vi "limit_array_size.vi"(10 "max size":i32, 11 "dbl array in":dbl[](array[numeric])) -> (3 "dbl array out":dbl[](array[numeric]))   [LabVIEW 2011]
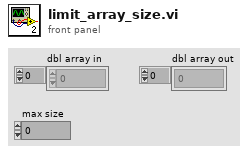
[diagram p1: front panel]
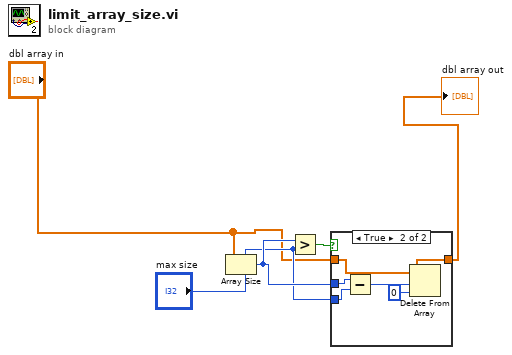
[diagram p0: block diagram]
diagram:
  n1 = Array Size(array="dbl array in") -> (size(s)=w5:i32)
  n2 = Greater?(x=w5, y="max size") -> (0:w1:bool)
  n3 = case shown="True" w1 {
    tunnel: "dbl array in" -> [w6 w12]
    tunnel: [w6 w11] -> w3
    tunnel: "max size" -> [_ w8]
    tunnel: w5 -> [_ w10]
    frame False {
    }
    frame True {
      n4 = Subtract(x=w10, y=w8) -> (x-y=w9:i32)
      n5 = Delete From Array(array=w12, length=w9, index=0) -> (array with subset deleted=w11:dbl[])  [unwired: 1 out]
    }
  }
  "dbl array out" <- w3
